vi "give_newline.vi"(11 "Array for writing":dbl[](array[numeric])) -> (3 "To file with newline":string)   [LabVIEW 2018]
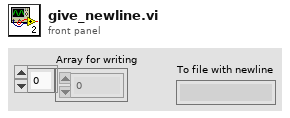
[diagram p1: front panel]
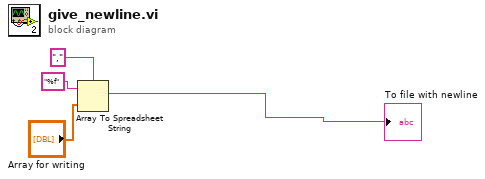
[diagram p0: block diagram]
diagram:
  n1 = Array To Spreadsheet String(delimiter (Tab)=",", array="Array for writing", 3:"%f") -> (spreadsheet string=→"To file with newline":string)
